vi "EX 4-2 Continuous Sampling.vi"() -> ()   [LabVIEW 2011, in "LabVIEW Interface for Arduino.lvlib"]
doc: "This VI shows an example of using the continuous aquisition mode on the Arduino to aquire analog input data from a single input pin. The user can set the sample rate for the aquisition when the VI is first run. The maximum aquisition speed of the Arduino is 5KHZ. While this mode is turned on executing other LIFA commands will corrupt analog data. To use other LIFA commands turn continuous mode off first."
uses:
  <vilib>/LabVIEW Interface for Arduino/LabVIEW Interface for Arduino.lvlib
panel:
  out "Waveform Chart":dbl[](graph)
  in  "Stop":bool
  in  "Sample Rate (HZ)":u16
  in  "Analog Input Pin":u8
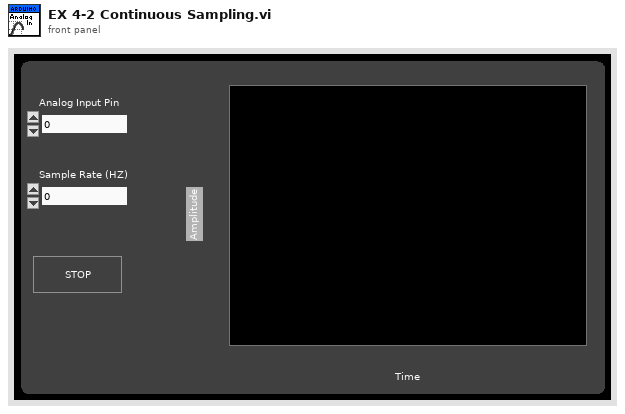
[diagram p1: front panel]
types:
  T1 = typedef "LabVIEW Interface for Arduino.lvlib/Arduino Resource.ctl" = cluster{"VISA resource":refnum<visa-resource-name>, "Board Type":T2, "Connection Type":enum8{"USB / Serial"}, "Bytes Per Packet (15)":u8}
  T2 = typedef "LabVIEW Interface for Arduino.lvlib/Board Type.ctl" = enum16{"Uno", "Dimuelanove w/Atmega 328", "Mega 2560"}
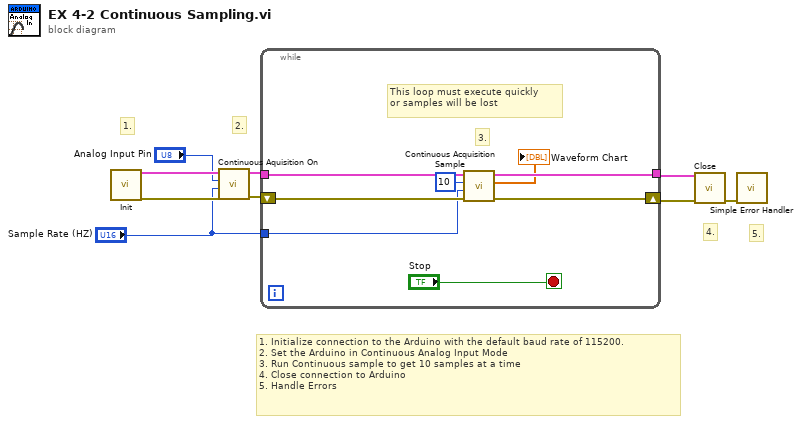
[diagram p0: block diagram]
diagram:
  # "5."
  # "4."
  # "2."
  # "1."
  # "1. Initialize connection to the Arduino with the default baud rate of 115200.\n2. Set the Arduino in Continuous Analog Input Mode\n3. Run Continuous sample to get 10 samples at a time\n4. Close connection to Arduino\n5. Handle Errors"
  n1 = call <vilib>:"Init.vi"() -> ("Arduino Resource"=w9:T1, "error out"=w2:errorcluster)  [unwired: 18 in]
  n2 = call <vilib>:"Continuous Aquisition On.vi"("error in"=w2, "Acquition Speed"="Sample Rate (HZ)", "Analog Input Pin"="Analog Input Pin", "Arduino Resource"=w9) -> ("error out"=w7:errorcluster, "Arduino Resource"=w8:T1)  [unwired: 6 in]
  n3 = while {
    tunnel: w8 -> [w16]
    tunnel: [w15] -> w6
    shift-right: [w14] -> w3
    shift-left: w7 -> [w13]
    tunnel: "Sample Rate (HZ)" -> [w10]
    stop <- "Stop" stop-if-true
    # "This loop must execute quickly\nor samples will be lost"
    # "3."
    n4 = call <vilib>:"Continuous Acquisition Sample.vi"("Arduino Resource"=w16, "Samples to Read"=u16 10, "Sample Rate (HZ)"=w10, "error in (no error)"=w13) -> ("Arduino Resource"=w15:T1, "Data"=→"Waveform Chart":dbl[], "error out"=w14:errorcluster)  [unwired: 4 in]
  }
  n5 = call <vilib>:"Close.vi"("Arduino Resource"=w6, "error in"=w3) -> ("error out"=w5:errorcluster)  [unwired: 13 in]
  n6 = call <vilib>:"Simple Error Handler.vi"("error in (no error)"=w5) -> ()  [unwired: 4 in, 5 out]
